vi "Read Measurement (Adjacent Channel Power).vi"(0 "VISA resource name":refnum<visa-resource-name>, 5 "ACP Carrier Number (1)":i32=1, 7 "ACP Method (1:EXE)":i32(ring)=1 items=["No Parameter", "EXE", "MOD", "TOTAL", "INBAND", "BOTH SIDES", "Number"], 11 "error in (no error)":errorcluster) -> (4 "VISA resource name out":refnum<visa-resource-name>, 6 "ACP Measurement":T1, 15 "error out":errorcluster)   [LabVIEW 2020, in "Anritsu Signal Analyzer Series.lvlib"]
doc: "Reads ACP measurement data"
uses:
  Anritsu Signal Analyzer Series.lvlib
panel:
  # "dBm/"
  # "Hz"
  # "dBm"
  # "dBc"
  # "dBm"
  # "dBc"
  # "dBm"
  # "dBc"
  # "dBm"
  # "dBc"
  # "dBm"
  # "dBc"
  # "dBm"
  # "dBc"
  # "dBm"
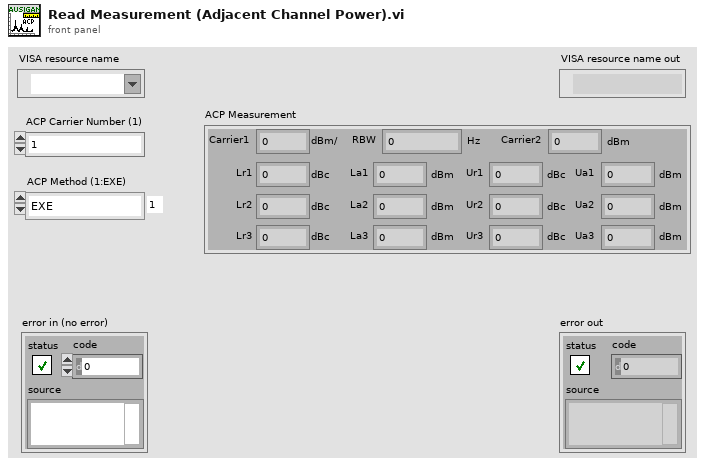
[diagram p1: front panel]
types:
  T1 = cluster{"Carrier1":dbl, "RBW":dbl, "Lr1":dbl, "La1":dbl, "Ur1":dbl, "Ua1":dbl, "Lr2":dbl, "La2":dbl, "Ur2":dbl, "Ua2":dbl, "Lr3":dbl, "La3":dbl, "Ur3":dbl, "Ua3":dbl, "Carrier2":dbl}
  T2 = cluster{"[0]":dbl, "[1]":dbl, "[2]":dbl, "[3]":dbl, "[4]":dbl, "[5]":dbl, "[6]":dbl, "[7]":dbl, "[8]":dbl, "[9]":dbl, "[10]":dbl, "[11]":dbl, "[12]":dbl, "[13]":dbl, "[14]":dbl}
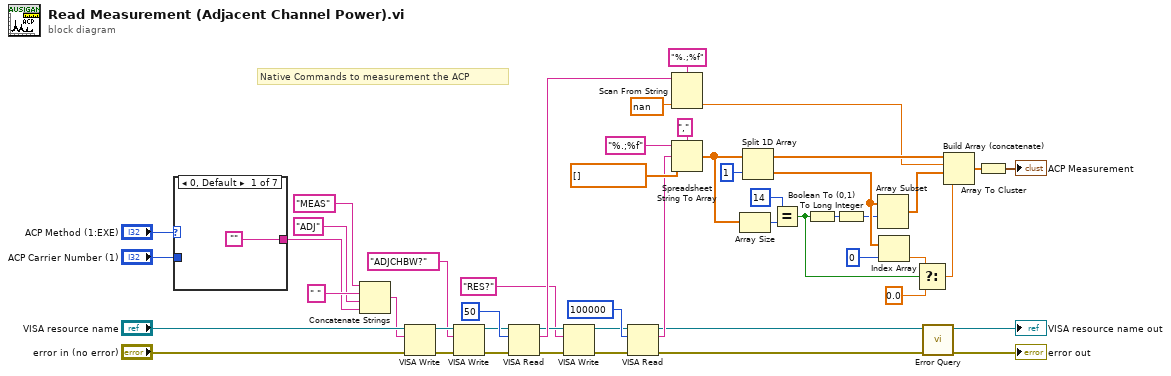
[diagram p0: block diagram]
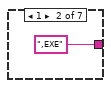
[diagram p2: hidden frame]
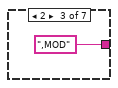
[diagram p3: hidden frame]
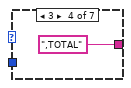
[diagram p4: hidden frame]
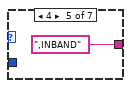
[diagram p5: hidden frame]
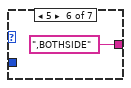
[diagram p6: hidden frame]
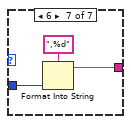
[diagram p7: hidden frame]
diagram:
  # "Native Commands to measurement the ACP"
  n1 = case shown="0, Default" "ACP Method (1:EXE)" {
    tunnel: ["" ("_Case1") ",EXE" ("_Case0") ",MOD" ("_Case1") ",TOTAL" ("_Case1") ",INBAND" ("_Case1") ",BOTHSIDE" ("_Case1") w57] -> w37
    tunnel: "ACP Carrier Number (1)" -> [_ _ _ _ _ _ w56]
    frame 0, Default {
    }
    frame 1 {
    }
    frame 2 {
    }
    frame 3 {
    }
    frame 4 {
    }
    frame 5 {
    }
    frame 6 {
      n2 = Format Into String(format string=",%d" ("_Case1"), w56) -> (resulting string=w57:string)  [unwired: 2 in, 1 out]
    }
  }
  n3 = Concatenate Strings("MEAS" ("_CommandSet"), " " ("string"), "ADJ", w37) -> (w36:string)
  n4 = VISA Write(VISA resource name="VISA resource name", write buffer=w36, error in (no error)="error in (no error)") -> (VISA resource name out=w28:refnum<visa-resource-name>, error out=w27:errorcluster)  [unwired: 1 out]
  n5 = VISA Write(VISA resource name=w28, write buffer="ADJCHBW?" ("_CommandGet"), error in (no error)=w27) -> (VISA resource name out=w30:refnum<visa-resource-name>, error out=w31:errorcluster)  [unwired: 1 out]
  n6 = VISA Read(VISA resource name=w30, byte count=u32 50 ("byte count (0)"), error in (no error)=w31) -> (VISA resource name out=w20:refnum<visa-resource-name>, read buffer=w33:string, error out=w19:errorcluster)  [unwired: 1 out]
  n7 = VISA Write(VISA resource name=w20, write buffer="RES?" ("_Command"), error in (no error)=w19) -> (VISA resource name out=w21:refnum<visa-resource-name>, error out=w22:errorcluster)  [unwired: 1 out]
  n8 = VISA Read(VISA resource name=w21, byte count=u32 100000 ("byte count (0)"), error in (no error)=w22) -> (VISA resource name out=w16:refnum<visa-resource-name>, read buffer=w18:string, error out=w17:errorcluster)  [unwired: 1 out]
  n9 = Scan From String(format string="%.;%f" ("Format String"), input string=w33, default 1=nan ("_Default")) -> (output 1=w13:dbl)  [unwired: 2 in, 3 out]
  n10 = Spreadsheet String To Array(delimiter (Tab)=",", format string="%.;%f", spreadsheet string=w18, array type (2D Dbl)=dbl[] [] ("Values")) -> (array=w12:dbl[])
  n11 = Array Size(array=w12) -> (size(s)=w11:i32)
  n12 = Split 1D Array(array=w12, index=1 ("Žw•W")) -> (first subarray=w41:dbl[], second subarray=w7:dbl[])
  n13 = Equal?(x=14, y=w11) -> (x = y?=w4:bool)
  n14 = Boolean To (0,1)(Boolean=w4) -> (0, 1=w8:i16)
  n15 = To Long Integer(number=w8) -> (32bit integer=w1:i32)
  n16 = Array Subset(array=w7, index=w1) -> (w9:dbl[])  [unwired: 1 in]
  n17 = Index Array(array=w7, index=0) -> (element=w5:dbl)
  n18 = Select(t=w5, s=w4, f=0.0) -> (s? t:f=w3:dbl)
  n19 = call "Error Query.vi"("error in (no error)"=w17, "VISA resource name"=w16) -> ("error out"=→"error out":errorcluster, "VISA resource name out"=→"VISA resource name out":refnum<visa-resource-name>)  [unwired: 6 in, 2 out]
  n20 = Build Array (concatenate)(w41, w13, w9, w3) -> (w40:dbl[])
  n21 = Array To Cluster(array=w40) -> (cluster=→"ACP Measurement":T2)
